vi "PH_PILS.ProcEvents.vi"(0 "i ref in":refnum<vi>, 5 "error in (no error)":errorcluster) -> (14 "i ref out":refnum<vi>, 19 "error out":errorcluster)   [LabVIEW 2014, in "PH_PILS.lvlib"]
doc: "This method is used to define the events the object will listen to. Add your own events here."
uses:
  PH_PILS.lvlib
  PH_Common/DIM/PH_DIM.Event Declarer.ctl
  PH_Beckhoff_PP_Control/PH_Beckhoff_PP_Control.PP Mercury Tags.ctl
  CSCore/BaseProcess/BaseProcess.lvlib
  PH_Common/PH_Common.lvlib
  PH_Beckhoff_PP_Control/PH_Beckhoff_PP_Control.lvlib
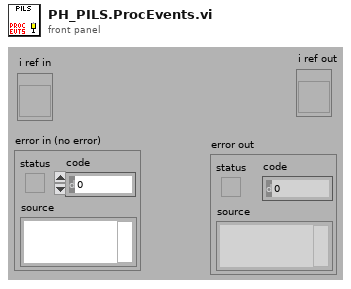
[diagram p1: front panel]
types:
  T1 = typedef "PH_Common.lvlib/PH_DIM.Event Declarer.ctl" = cluster{"Service Name":string, "Selector":string}
  T2 = typedef "PH_Beckhoff_PP_Control.lvlib/PH_Beckhoff_PP_Control.PP Mercury Tags.ctl" = enum16{"Device-on", "Alarm", "on-since", "Concentration", "Status"}
  T3 = typedef "PH_PILS.lvlib/PH_PILS.i attribute.ctl" = cluster{"Boolean":cluster{"GUI Ref":refnum<vi>, "Status":i32}[], "GUI Refs Exp. Shutters":cluster{"1":refnum<vi>, "2":refnum<vi>, "3":refnum<vi>, "4":refnum<vi>}, "Tristate2Run GUI Refs":refnum<vi>[], "EO-Likes":cluster{"GUI Ref":refnum<vi>, "Status":i32}[], "Operation Mode":cluster{"Operation Mode":T4, "GUI":cluster{"Ref State":refnum<vi>, "Ref":refnum<vi>}, "Servicemode":cluster{"Tagname":string, "Status":i32}, "Labormode":cluster{"Tagname":string, "Status":i32}, "Searchmode":cluster{"Tagname":string, "Status":i32}, "Shotmode":cluster{"Tagname":string, "Status":i32}}, "Submode":cluster{"Submode":T5, "GUI":cluster{"Ref State":refnum<vi>, "Ref":refnum<vi>}, "Submode":cluster{"Tagname":string, "Status":i32}}, "Experiment":cluster{"Experiment":enum16{"unknown", "intern", "4 (Z6)", "3", "2", "1"}, "GUI":cluster{"Ref State":refnum<vi>, "Ref":refnum<vi>}, "intern":cluster{"Tagname":string, "Status":i32}, "Exp 4":cluster{"Tagname":string, "Status":i32}, "Exp 3":cluster{"Tagname":string, "Status":i32}, "Exp 2":cluster{"Tagname":string, "Status":i32}, "Exp 1":cluster{"Tagname":string, "Status":i32}}, "TristateNormal":cluster{"GUI Ref":refnum<vi>, "Status":i32}[], "Door Tags":cluster{"GUI Ref":refnum<vi>, "Status":i32}[], "GUIlessTags":cluster{"Name":string, "Status":i32}[], "Beamline GUI Refs":refnum<vi>[], "Special Boolean":cluster{"GUI Ref":refnum<vi>, "Status":i32}[], "Laserpower":cluster{"GUI Ref":refnum<vi>, "Status":i32}[], "Shutter":cluster{"GUI Ref":refnum<vi>, "Status":i32}[], "Tristate EO Like":cluster{"GUI Ref":refnum<vi>, "Status":i32}[], "PP":cluster{"GUI Ref":refnum<vi>, "Status":i32, "Head Ref":refnum<vi>, "Slider Ref":refnum<vi>}[], "Switch Knobs":cluster{"GUI Ref":refnum<vi>, "Status":i32}[], "Latch Knob GUI Refs":refnum<vi>[], "FailureCounter":i32, "Enabled Status":cluster{"Laser":i32, "PreAmp":i32, "MainAmp":i32}, "Mercury":refnum<vi>, "Instance Rods":string, "Logfile":path, "Beckhoff-Instance Internal":string, "Beckhoff-Instance External":string, "Enabling Rights":cluster{"Name":string, "Password":string, "PA?":bool, "MA?":bool, "Exp?":bool}[]}
  T4 = typedef "PH_PILS.lvlib/PH_PILS.Operation Mode.ctl" = enum16{"unknown", "Service", "Labor", "Search", "Shot"}
  T5 = typedef "PH_PILS.lvlib/PH_PILS.Submode.ctl" = enum16{"unknown", "HV-Normal", "HV-Test"}
  T6 = cluster{"GUI Ref":refnum<vi>, "Status":i32, "Head Ref":refnum<vi>, "Slider Ref":refnum<vi>}[]
  T7 = typedef "BaseProcess.lvlib/BaseProcess.event definition.ctl" = cluster{"CAEEvtDef":T8, "Data Descriptor":T9}
  T8 = typedef "CAEObj.lvlib/CAEObj.event definition.ctl" = cluster{"URL":string, "enable":bool, "ignoreResID":bool}
  T9 = typedef "BaseProcess.lvlib/BaseProcess.descriptor string definition.ctl" = string
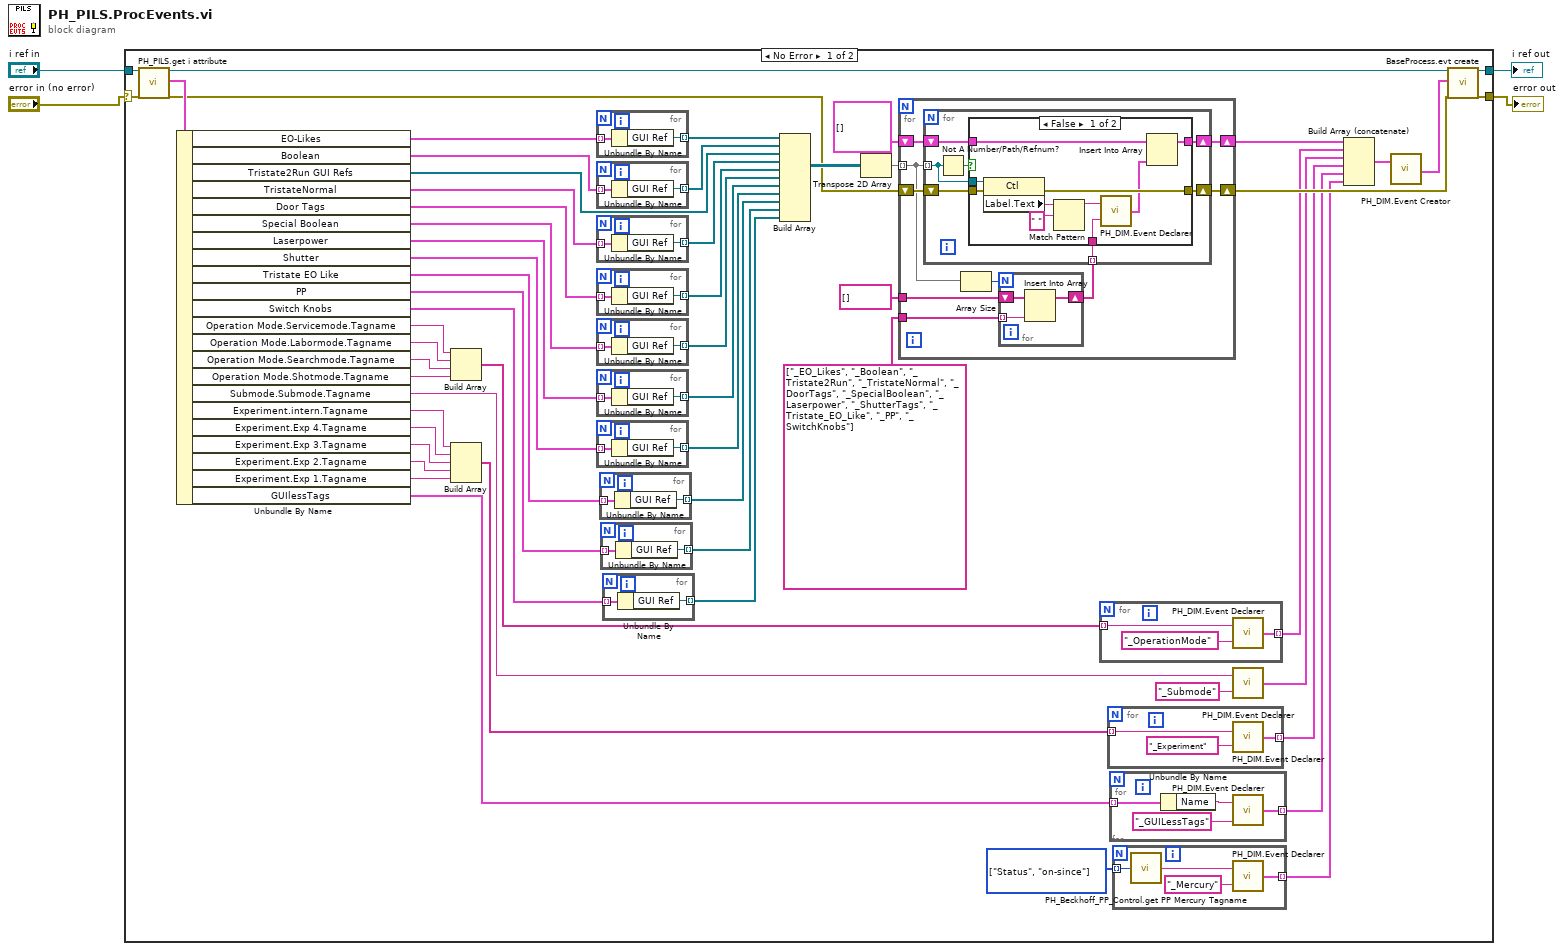
[diagram p0: block diagram]
diagram:
  n1 = case shown="No Error" "error in (no error)" {
    selector: "error in (no error)" -> [w56 w128]
    tunnel: "i ref in" -> [w58 w127]
    tunnel: [w61 w127] -> w3
    tunnel: [w60 w128] -> w2
    frame No Error {
      w6 = T2[] [enum."Status", enum."on-since"] items=["Device-on", "Alarm", "on-since", "Concentration", "Status"]
      n2 = call "PH_PILS.get i attribute.vi"("i ref in"=w58, "error in (no error)"=w56) -> ("i ref out"=w57:refnum<vi>, "i attribute"=w59:T3, "error out"=w23:errorcluster)  [unwired: 15 in]
      n3 = Unbundle By Name(w59) -> ("EO-Likes"=w48:cluster{"GUI Ref":refnum<vi>, "Status":i32}[], "Boolean"=w54:cluster{"GUI Ref":refnum<vi>, "Status":i32}[], "Tristate2Run GUI Refs"=w49:refnum<vi>[], "TristateNormal"=w32:cluster{"GUI Ref":refnum<vi>, "Status":i32}[], "Door Tags"=w30:cluster{"GUI Ref":refnum<vi>, "Status":i32}[], "Special Boolean"=w27:cluster{"GUI Ref":refnum<vi>, "Status":i32}[], "Laserpower"=w25:cluster{"GUI Ref":refnum<vi>, "Status":i32}[], "Shutter"=w11:cluster{"GUI Ref":refnum<vi>, "Status":i32}[], "Tristate EO Like"=w18:cluster{"GUI Ref":refnum<vi>, "Status":i32}[], "PP"=w15:T6, "Switch Knobs"=w13:cluster{"GUI Ref":refnum<vi>, "Status":i32}[], "Operation Mode.Servicemode.Tagname"=w46:string, "Operation Mode.Labormode.Tagname"=w45:string, "Operation Mode.Searchmode.Tagname"=w44:string, "Operation Mode.Shotmode.Tagname"=w43:string, "Submode.Submode.Tagname"=w10:string, "Experiment.intern.Tagname"=w39:string, "Experiment.Exp 4.Tagname"=w38:string, "Experiment.Exp 3.Tagname"=w37:string, "Experiment.Exp 2.Tagname"=w36:string, "Experiment.Exp 1.Tagname"=w35:string, "GUIlessTags"=w7:cluster{"Name":string, "Status":i32}[])
      n4 = Build Array(w46, w45, w44, w43) -> (w41:string[])
      n5 = Build Array(w39, w38, w37, w36, w35) -> (w34:string[])
      n6 = for {
        tunnel: w48 -> [w93] mode=indexing
        tunnel: [w92] -> w47 mode=indexing
        n7 = Unbundle By Name(w93) -> ("GUI Ref"=w92:refnum<vi>)
      }
      n8 = for {
        tunnel: w54 -> [w126] mode=indexing
        tunnel: [w125] -> w51 mode=indexing
        n9 = Unbundle By Name(w126) -> ("GUI Ref"=w125:refnum<vi>)
      }
      n10 = for {
        tunnel: w32 -> [w85] mode=indexing
        tunnel: [w84] -> w31 mode=indexing
        n11 = Unbundle By Name(w85) -> ("GUI Ref"=w84:refnum<vi>)
      }
      n12 = for {
        tunnel: w30 -> [w83] mode=indexing
        tunnel: [w82] -> w29 mode=indexing
        n13 = Unbundle By Name(w83) -> ("GUI Ref"=w82:refnum<vi>)
      }
      n14 = for {
        tunnel: w27 -> [w77] mode=indexing
        tunnel: [w76] -> w26 mode=indexing
        n15 = Unbundle By Name(w77) -> ("GUI Ref"=w76:refnum<vi>)
      }
      n16 = for {
        tunnel: w25 -> [w75] mode=indexing
        tunnel: [w74] -> w24 mode=indexing
        n17 = Unbundle By Name(w75) -> ("GUI Ref"=w74:refnum<vi>)
      }
      n18 = for {
        tunnel: w11 -> [w73] mode=indexing
        tunnel: [w72] -> w19 mode=indexing
        n19 = Unbundle By Name(w73) -> ("GUI Ref"=w72:refnum<vi>)
      }
      n20 = for {
        tunnel: w18 -> [w71] mode=indexing
        tunnel: [w70] -> w17 mode=indexing
        n21 = Unbundle By Name(w71) -> ("GUI Ref"=w70:refnum<vi>)
      }
      n22 = for {
        tunnel: w15 -> [w69] mode=indexing
        tunnel: [w68] -> w14 mode=indexing
        n23 = Unbundle By Name(w69) -> ("GUI Ref"=w68:refnum<vi>)
      }
      n24 = for {
        tunnel: w13 -> [w67] mode=indexing
        tunnel: [w66] -> w12 mode=indexing
        n25 = Unbundle By Name(w67) -> ("GUI Ref"=w66:refnum<vi>)
      }
      n26 = Build Array(w47, w51, w49, w31, w29, w26, w24, w19, w17, w14, w12) -> (w53:refnum<vi>[][])
      n27 = Transpose 2D Array(2D array=w53) -> (transposed array=w20:refnum<vi>[][])
      n28 = for {
        tunnel: w20 -> [w97] mode=indexing
        shift-right: [w101] -> w55
        shift-left: w23 -> [w102]
        shift-right: [w99] -> w16
        shift-left: T1[] [] -> [w100]
        tunnel: string[] ["_EO_Likes", "_Boolean", "_Tristate2Run", "_TristateNormal", "_DoorTags", "_SpecialBoolean", "_Laserpower", "_ShutterTags", "_Tristate_EO_Like", "_PP", "_SwitchKnobs"] -> [w96]
        tunnel: string[] [] -> [w95]
        n29 = Array Size(array=w97) -> (size(s)=w98:i32)
        n30 = for {
          N: w98 -> [_]
          tunnel: w96 -> [w105] mode=indexing
          shift-right: [w104] -> w94
          shift-left: w95 -> [w103]
          n31 = Insert Into Array(array=w103, new element=w105) -> (w104:string[])  [unwired: 1 in]
        }
        n32 = for {
          tunnel: w97 -> [w110] mode=indexing
          tunnel: w94 -> [w108] mode=indexing
          shift-right: [w111] -> w101
          shift-left: w102 -> [w112]
          shift-right: [w106] -> w99
          shift-left: w100 -> [w107]
          n33 = Not A Number/Path/Refnum?(number/path/refnum=w110) -> (NaN/Path/Refnum?=w109:bool)
          n34 = case shown="False" w109 {
            tunnel: [w122 w124] -> w111
            tunnel: w112 -> [w121 w124]
            tunnel: w110 -> [w120 _]
            tunnel: w108 -> [w115 _]
            tunnel: w107 -> [w119 w123]
            tunnel: [w118 w123] -> w106
            frame False {
              n35 = property class="Ctl"(reference=w120, error in=w121) -> (error out=w122:errorcluster, "Label.Text"=w116:string)  [unwired: 1 out]
              n36 = Match Pattern(string=w116, regular expression=" ") -> (before substring=w114:string)  [unwired: 1 in, 3 out]
              n37 = call "PH_DIM.Event Declarer.vi"("Selector"=w115, "Service Name"=w114) -> ("declared DIM Event"=w113:T1)
              n38 = Insert Into Array(array=w119, new element=w113) -> (w118:T1[])  [unwired: 1 in]
            }
            frame True {
            }
          }
        }
      }
      n39 = for {
        tunnel: w41 -> [w91] mode=indexing
        tunnel: [w90] -> w40 mode=indexing
        n40 = call "PH_DIM.Event Declarer.vi"("Selector"="_OperationMode", "Service Name"=w91) -> ("declared DIM Event"=w90:T1)
      }
      n41 = for {
        tunnel: w34 -> [w88] mode=indexing
        tunnel: [w87] -> w33 mode=indexing
        n42 = call "PH_DIM.Event Declarer.vi"("Selector"="_Experiment", "Service Name"=w88) -> ("declared DIM Event"=w87:T1)
      }
      n43 = for {
        tunnel: [w81] -> w28 mode=indexing
        tunnel: w7 -> [w78] mode=indexing
        n44 = Unbundle By Name(w78) -> ("Name"=w79:string)
        n45 = call "PH_DIM.Event Declarer.vi"("Selector"="_GUILessTags", "Service Name"=w79) -> ("declared DIM Event"=w81:T1)
      }
      n46 = for {
        tunnel: w6 -> [w65] mode=indexing
        tunnel: [w63] -> w5 mode=indexing
        n47 = call "PH_Beckhoff_PP_Control.get PP Mercury Tagname.vi"("PP Mercury Tag"=w65) -> ("PP Mercury Tagname"=w64:string)
        n48 = call "PH_DIM.Event Declarer.vi"("Selector"="_Mercury", "Service Name"=w64) -> ("declared DIM Event"=w63:T1)
      }
      n49 = call "PH_DIM.Event Declarer.vi"("Selector"="_Submode", "Service Name"=w10) -> ("declared DIM Event"=w8:T1)
      n50 = Build Array (concatenate)(w16, w40, w8, w33, w28, w5) -> (w42:T1[])
      n51 = call "PH_DIM.Event Creator.vi"("Trendmessage Services"=w42) -> ("DIM Service Events"=w50:T7[])  [unwired: 18 in]
      n52 = call "BaseProcess.evt create.vi"("i ref in"=w57, "newEvents"=w50, "error in (no error)"=w55) -> ("i ref out"=w61:refnum<vi>, "error out"=w60:errorcluster)  [unwired: 13 in, 2 out]
    }
    frame Error {
    }
  }
  "i ref out" <- w3
  "error out" <- w2
